vi "Asynchronous Random Number Generator.vi"(11 "Queue in":refnum<queue>) -> ()   [LabVIEW 2017]
doc: "A basic asynchronous loop which will return a random number after 100ms of a request. It will resolve the future to an error if the random number is less than 0.1\n\nIt supports promises and notifiers to support a comparison."
uses:
  Command Queue Data.ctl
  Futures/Promise/Promise.lvclass
  49ca4dfa-3b5a-4d33-b042-d93a1aeda566.vi
  <vilib>/Utility/error.llb/Error Cluster From Error Code.vi
  <vilib>/ErrorRing/Error Ring.xnode
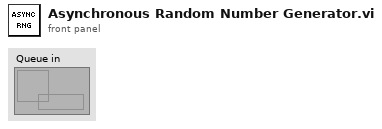
[diagram p1: front panel]
types:
  T1 = typedef "Command Queue Data.ctl" = cluster{"Promise":refnum<class "Promise.lvclass">, "notifier":refnum<notifier>}
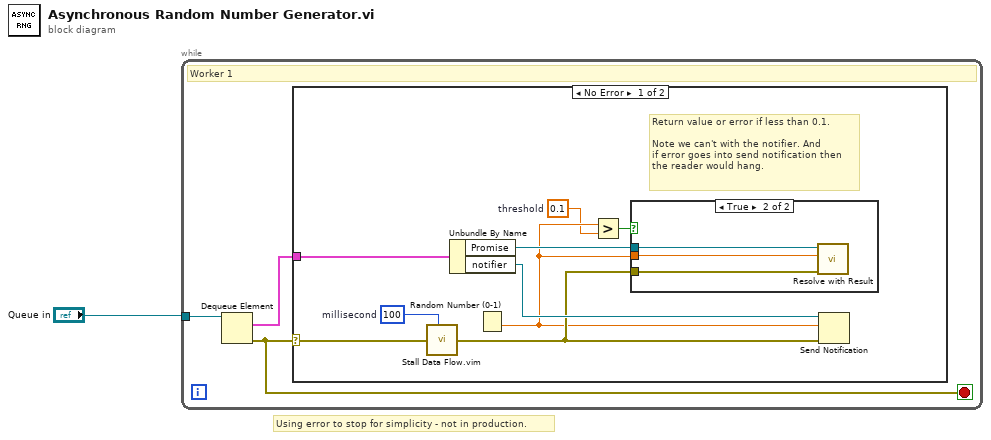
[diagram p0: block diagram]
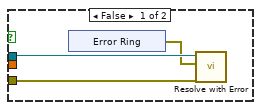
[diagram p2: hidden frame]
diagram:
  # "Using error to stop for simplicity - not in production."
  n1 = while {
    tunnel: "Queue in" -> [w4]
    stop <- w2 stop-if-true
    # "Worker 1"
    n2 = Dequeue Element(queue=w4) -> (element=w3:T1, error out=w2:errorcluster)  [unwired: 2 in, 2 out]
    n3 = case shown="No Error" w2 {
      selector: w2 -> [w12 _]
      tunnel: w3 -> [w13 _]
      frame No Error {
        w6 = 0.1  # threshold
        w8 = u32 100  # millisecond
        # "Return value or error if less than 0.1.\n\nNote we can't with the notifier. And\nif error goes into send notification then\nthe reader would hang."
        n4 = call "Stall Data Flow.vim"("value in"=w12, "milliseconds to wait"=w8) -> ("value out"=w9:errorcluster)  [unwired: 1 out]
        n5 = Unbundle By Name(w13) -> ("Promise"=w10:refnum<class "Promise.lvclass">, "notifier"=w11:refnum<notifier>)
        n6 = Random Number (0-1)() -> (number: 0 to 1=w7:dbl)
        n7 = Greater?(x=w7, y=w6) -> (0:w5:bool)
        n8 = case shown="True" w5 {
          tunnel: w10 -> [w16 w24]
          tunnel: w9 -> [w15 w23]
          tunnel: w7 -> [_ w22]
          frame False {
            n9 = xnode "Error Ring"() -> ("error out"=w14:errorcluster)
            n10 = call "Resolve with Error.vi"("error in (no error)"=w15, "Result"=w14, "Promise in"=w16) -> ()  [unwired: 8 in, 1 out]
          }
          frame True {
            n11 = call "Resolve with Result.vi"("error in (no error)"=w23, "Result"=w22, "Promise in"=w24) -> ()  [unwired: 8 in, 1 out]
          }
        }
        n12 = Send Notification(notification=w7, notifier=w11, error in (no error)=w9) -> ()  [unwired: 2 out]
      }
      frame Error {
      }
    }
  }
